vi "PriceData Test.vi"(8 "error in":errorcluster, 11 "IED Test in":refnum<class "IED Test.lvclass">) -> (0 "error out":errorcluster, 2 "Test Result":T1=enum."Success", 3 "IED Test out":refnum<class "IED Test.lvclass">)   [LabVIEW 2018, in "IED Test Framework.lvlib" / "IED Test.lvclass"]
uses:
  IED Test.lvclass
  C:/Program Files (x86)/National Instruments/LabVIEW 2018/vi.lib/ActorFramework/Actor/Actor.lvclass
  C:/Users/Administrator/Desktop/2018LabVIEW EMS/EMS Generic Actor/EMS Generic/EMS Generic.lvclass
  Controls/Test Result.ctl
  <vilib>/ORNL/CSEISMIC DDS/CSEISMIC DDS Base/Data Types/Controls/DeviceClass Selector.ctl
  PriceData Actor/PriceData/PriceData.lvclass
  C:/Users/Administrator/Desktop/2018LabVIEW EMS/IED Actors/Device DDS Communications Framework/Device DDS Communications/Device DDS Communications.lvclass
  <vilib>/ORNL/CSEISMIC DDS/CSEISMIC DDS Base/CSEISMIC DDS.lvclass/CSEISMIC DDS.ctl
  <vilib>/ORNL/CSEISMIC DDS/CSEISMIC DDS Base/Data Types/Controls/DeviceID.ctl
  <vilib>/ActorFramework/Message Enqueuer/Message Enqueuer.lvclass/Message Enqueuer.ctl
  <vilib>/ORNL/CSEISMIC DDS/CSEISMIC DDS Base/Accessors/Write DDS Reference.vi
  <vilib>/ORNL/CSEISMIC DDS/CSEISMIC DDS Base/Accessors/Read DDS Reference.vi
  <vilib>/ActorFramework/Message Enqueuer/Enqueue.vi
  <vilib>/ORNL/CSEISMIC DDS/DDS Writer/DDS Writer.lvclass
  C:/Program Files (x86)/National Instruments/LabVIEW 2018/vi.lib/ORNL/CSEISMIC DDS/CSEISMIC DDS Base/CSEISMIC DDS.lvclass
  <vilib>/ActorFramework/Stop Msg/Stop Msg.lvclass
  C:/Program Files (x86)/National Instruments/LabVIEW 2018/vi.lib/ActorFramework/Message/Message.lvclass
  <vilib>/ORNL/CSEISMIC DDS/CSEISMIC DDS Base/Error Handler.vi
  <vilib>/ActorFramework/Message Priority Queue/Priority Enqueue.vi
  <vilib>/ORNL/CSEISMIC DDS/CSEISMIC DDS Base/CSEISMIC DDS.lvclass
  Device DDS Communications Framework/Device DDS Communications/Device DDS Communications.lvclass
  <vilib>/ActorFramework/Actor/Actor.lvclass
  EMS Generic Actor/EMS Generic/EMS Generic.lvclass
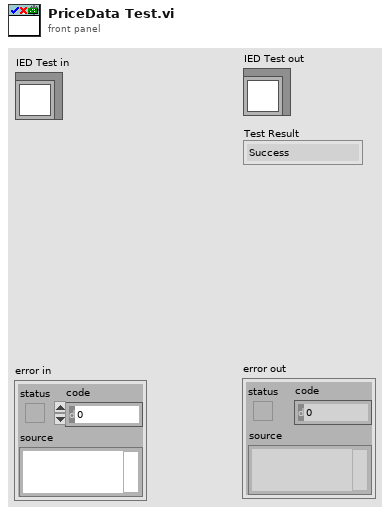
[diagram p1: front panel]
types:
  T1 = typedef "IED Test Framework.lvlib/IED Test.lvclass/Test Result.ctl" = enum16{"Invalid", "Success", "Failure", "Error", "Timeout"}
  T2 = typedef "CSEISMIC DDS.lvlib/CSEISMIC DDS.lvclass/DeviceID.ctl" = string
  T3 = typedef "CSEISMIC DDS.lvlib/CSEISMIC DDS.lvclass/DeviceClass Selector.ctl" = u16
  T4 = typedef "CSEISMIC DDS.lvlib/CSEISMIC DDS.lvclass/PriceData_RealTime.ctl" = cluster{"DeviceID":T2, "t0":dbl, "dt":dbl, "Price":dbl[]}
  T5 = typedef "CSEISMIC DDS.lvlib/CSEISMIC DDS.lvclass/PriceData_Demand.ctl" = cluster{"DeviceID":T2, "DemandCharge ($/kWh)":dbl, "Duration (hours)":dbl}
  T6 = typedef "CSEISMIC DDS.lvlib/CSEISMIC DDS.lvclass/PriceData_Energy.ctl" = cluster{"DeviceID":T2, "EnergyCharge ($/kWh)":dbl}
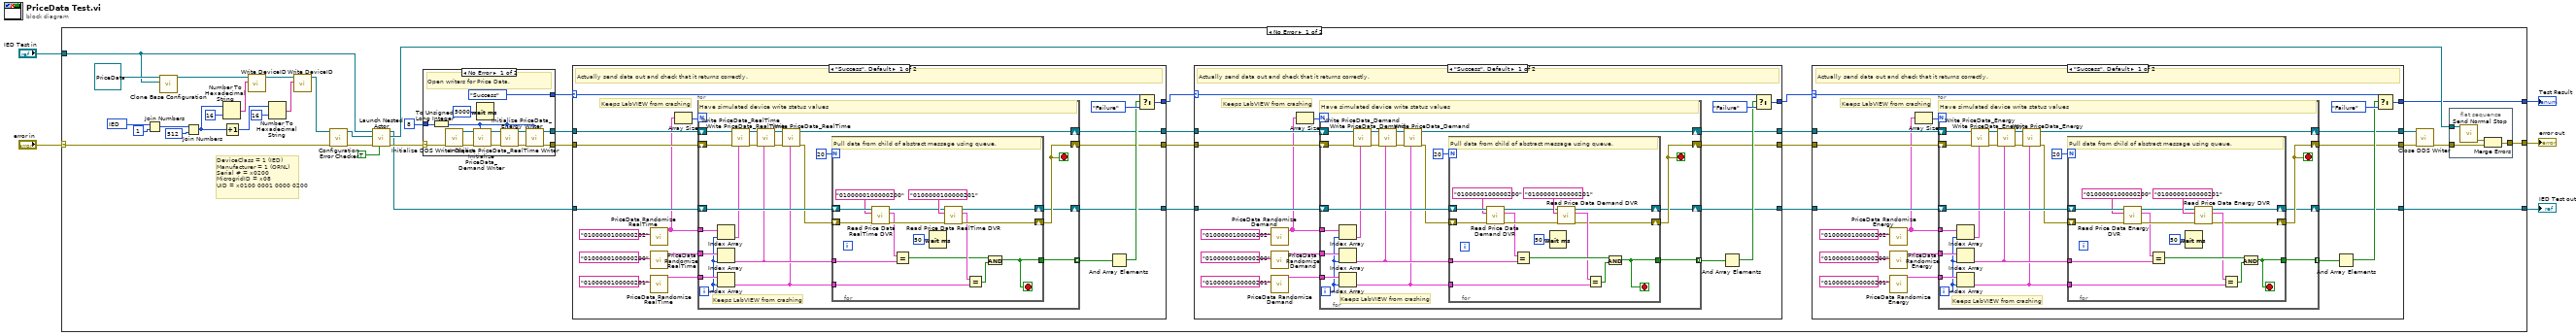
[diagram p0: block diagram]
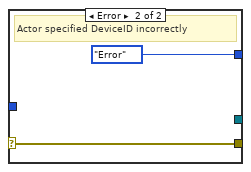
[diagram p5: hidden frame]
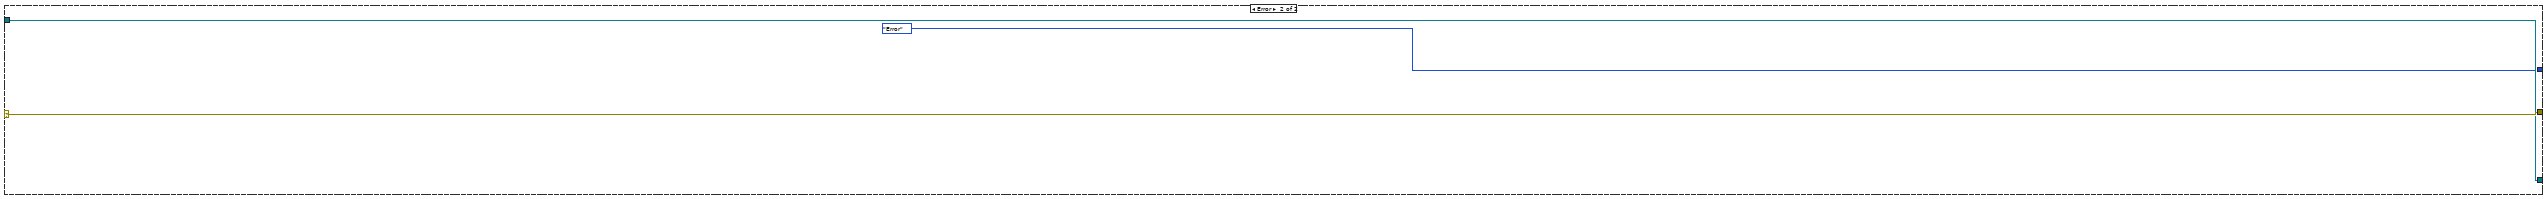
[diagram p6: hidden frame]
diagram:
  n1 = case shown="No Error" "error in" {
    selector: "error in" -> [w41 w241]
    tunnel: [w43 w241] -> w2
    tunnel: [w9 w240] -> w1
    tunnel: "IED Test in" -> [w6 w240]
    tunnel: [w13 Test_Result."Error" ("f")] -> w3
    frame No Error {
      w34 = T3 256 items=["Invalid"=0, "IED"=256, "DER"=512, "Relay"=768, "Meter"=1024, "Load"=1280, "Forecast"=1536, "Price"=1792, "Energy Storage"=513, "PV"=514, "Generator"=515, "Smart Relay"=769, "PCC"=770, "Smart Meter"=1025, "PMU"=1026, "HVAC"=1281] ("DeviceClass")
      # "DeviceClass = 1 (IED)\nManufacturer = 1 (ORNL)\nSerial # = x0200\nMicrogridID = x08\nUID = x0100 0001 0000 0200"
      n2 = Join Numbers(hi=w34, lo=u16 1 ("MicrogridID")) -> ((hi.lo)=w31:u32)
      n3 = call-dynamic "Clone Base Configuration.vi"("Source Object"=w6, "Target Object in"=refnum<class "PriceData.lvclass"> refnum ("PriceData Actor.lvlib:PriceData.lvclass")) -> ("Target Object out"=w7:refnum<class "PriceData.lvclass">)  [unwired: 9 in]
      n4 = Join Numbers(hi=w31, lo=u32 512 ("MicrogridID")) -> ((hi.lo)=w36:u64)
      n5 = Number To Hexadecimal String(1:i16 16 ("width (-)"), 2:w36) -> (0:w29:string)
      n6 = Increment(x=w36) -> (x+1=w38:u64)
      n7 = call-dynamic "Write DeviceID.vi"("DeviceID"=w29, "Device DDS Communications in"=w7) -> ("Device DDS Communications out"=w33:refnum<class "PriceData.lvclass">)  [unwired: 9 in]
      n8 = Number To Hexadecimal String(1:i16 16 ("width (-)"), 2:w38) -> (0:w39:string)
      n9 = call-dynamic "Write DeviceID.vi"("DeviceID"=w39, "Device DDS Communications in"=w33) -> ("Device DDS Communications out"=w19:refnum<class "PriceData.lvclass">)  [unwired: 9 in]
      n10 = call "Configuration Error Checker.vi"("error in"=w41, "Device DDS Communications in"=w19) -> ("error out"=w44:errorcluster, "Device DDS Communications out"=w42:refnum<class "PriceData.lvclass">)  [unwired: 8 in]
      n11 = call <vilib>:"Launch Nested Actor.vi"("Open Actor Core front panel? (F)"=TRUE, "error in (no error)"=w44, "Nested Actor"=w42, "Caller Actor in"=w6) -> ("error out"=w27:errorcluster, "Nested Actor's Enqueuer"=w40:refnum<class "Message Enqueuer.lvclass">, "Caller Actor out"=w10:refnum<class "IED Test.lvclass">)  [unwired: 5 in]
      n12 = case shown="No Error" w27 {
        selector: w27 -> [w234 w238]
        tunnel: [w228 w238] -> w24
        tunnel: u32 8 ("domain id") -> [w236 _]
        tunnel: [Test_Result."Success" ("Test Result in") Test_Result."Error" ("Test Result")] -> w26
        tunnel: [w225 _] -> w25
        frame No Error {
          # "Open writers for Price Data."
          n13 = To Unsigned Long Integer(number=w236) -> (unsigned 32bit integer=w224:u32)
          n14 = call <vilib>:"Initialize DDS Writer Object.vi"("error in"=w234) -> ("error out"=w233:errorcluster, "DDS Writer out"=w232:refnum<class "DDS Writer.lvclass">)  [unwired: 9 in]
          n15 = call <vilib>:"Initialize PriceData_Demand Writer.vi"("MicrogridID"=w224, "error in"=w233, "DDS Writer in"=w232) -> ("error out"=w230:errorcluster, "DDS Writer out"=w231:refnum<class "DDS Writer.lvclass">)  [unwired: 7 in]
          n16 = Wait (ms)(milliseconds to wait=u32 5000) -> ()  [unwired: 1 out]
          n17 = call <vilib>:"Initialize PriceData_Energy Writer.vi"("MicrogridID"=w224, "error in"=w230, "DDS Writer in"=w231) -> ("error out"=w226:errorcluster, "DDS Writer out"=w227:refnum<class "DDS Writer.lvclass">)  [unwired: 7 in]
          n18 = call <vilib>:"Initialize PriceData_RealTime Writer.vi"("MicrogridID"=w224, "error in"=w226, "DDS Writer in"=w227) -> ("error out"=w228:errorcluster, "DDS Writer out"=w225:refnum<class "DDS Writer.lvclass">)  [unwired: 7 in]
        }
        frame Error {
          # "Actor specified DeviceID incorrectly"
        }
      }
      n19 = case shown="\"Success\", Default" w26 {
        selector: w26 -> [w182 w222]
        tunnel: w25 -> [w183 w221]
        tunnel: w10 -> [w177 w220]
        tunnel: w24 -> [w178 w223]
        tunnel: [w180 w222] -> w21
        tunnel: [w176 w223] -> w22
        tunnel: [w174 w221] -> w23
        tunnel: [w167 w220] -> w12
        frame "Success", Default {
          # "Keeps LabVIEW from crashing"
          # "Actually send data out and check that it returns correctly."
          n20 = call "PriceData Randomize RealTime.vi"("DeviceID"=T2 "0100000100000202" ("(hi.lo)")) -> ("ForecastData_Long Array out"=w173:T4[])  [unwired: 10 in]
          n21 = call "PriceData Randomize RealTime.vi"("DeviceID"=T2 "0100000100000200" ("(hi.lo)")) -> ("ForecastData_Long Array out"=w168:T4[])  [unwired: 10 in]
          n22 = call "PriceData Randomize RealTime.vi"("DeviceID"=T2 "0100000100000201" ("(hi.lo)")) -> ("ForecastData_Long Array out"=w169:T4[])  [unwired: 10 in]
          n23 = Array Size(array=w173) -> (size(s)=w175:i32)
          n24 = for {
            N: w175 -> [_]
            shift-right: [w200] -> w174
            shift-left: w183 -> [w203]
            tunnel: w173 -> [w196]
            tunnel: w169 -> [w191]
            tunnel: w168 -> [w192]
            shift-right: [w193] -> w176
            shift-left: w178 -> [w199]
            shift-right: [w187] -> w167
            shift-left: w177 -> [w195]
            tunnel: [w184] -> w166 mode=indexing
            i -> [w189]
            stop <- w193 stop-if-true
            # "Keeps LabVIEW from crashing"
            # "Have simulated device write status values"
            n25 = Index Array(array=w196, index=w189) -> (element=w188:T4)
            n26 = Index Array(array=w192, index=w189) -> (element=w186:T4)
            n27 = Index Array(array=w191, index=w189) -> (element=w185:T4)
            n28 = call <vilib>:"Write PriceData_RealTime.vi"("PriceData_RealTime"=w188, "error in"=w199, "DDS Writer in"=w203) -> ("error out"=w198:errorcluster, "DDS Writer out"=w202:refnum<class "DDS Writer.lvclass">)  [unwired: 7 in]
            n29 = call <vilib>:"Write PriceData_RealTime.vi"("PriceData_RealTime"=w186, "error in"=w198, "DDS Writer in"=w202) -> ("error out"=w197:errorcluster, "DDS Writer out"=w201:refnum<class "DDS Writer.lvclass">)  [unwired: 7 in]
            n30 = call <vilib>:"Write PriceData_RealTime.vi"("PriceData_RealTime"=w185, "error in"=w197, "DDS Writer in"=w201) -> ("error out"=w194:errorcluster, "DDS Writer out"=w200:refnum<class "DDS Writer.lvclass">)  [unwired: 7 in]
            n31 = for {
              N: 20 -> [_]
              shift-right: [w212] -> w193
              shift-left: w194 -> [w218]
              shift-right: [w213] -> w187
              shift-left: w195 -> [w219]
              tunnel: w186 -> [w211]
              tunnel: w185 -> [w209]
              tunnel: [w205] -> w184
              stop <- w205 stop-if-true
              # "Pull data from child of abstract message using queue."
              n32 = call "Read Price Data RealTime DVR.vi"("error in"=w218, "DeviceID"=T2 "0100000100000200" ("(hi.lo)"), "EMS Generic in"=w219) -> ("error out"=w214:errorcluster, "PriceData_RealTime"=w210:T4, "EMS Generic out"=w215:refnum<class "IED Test.lvclass">)  [unwired: 5 in, 1 out]
              n33 = Equal?(x=w210, y=w211) -> (x = y?=w207:bool)
              n34 = Wait (ms)(milliseconds to wait=u32 50) -> ()  [unwired: 1 out]
              n35 = call "Read Price Data RealTime DVR.vi"("error in"=w214, "DeviceID"=T2 "0100000100000201" ("(hi.lo)"), "EMS Generic in"=w215) -> ("error out"=w212:errorcluster, "PriceData_RealTime"=w208:T4, "EMS Generic out"=w213:refnum<class "IED Test.lvclass">)  [unwired: 5 in, 1 out]
              n36 = Equal?(x=w208, y=w209) -> (x = y?=w206:bool)
              n37 = And(x=w207, y=w206) -> (x .and. y?=w205:bool)
            }
          }
          n38 = And Array Elements(Boolean array=w166) -> (logical AND=w179:bool)
          n39 = Select(t=w182, s=w179, f=Test_Result."Failure") -> (s? t:f=w180:T1)
        }
        frame "Error" {
        }
      }
      n40 = case shown="\"Success\", Default" w21 {
        selector: w21 -> [w124 w164]
        tunnel: w23 -> [w125 w163]
        tunnel: w12 -> [w119 w162]
        tunnel: w22 -> [w120 w165]
        tunnel: [w122 w164] -> w16
        tunnel: [w118 w165] -> w17
        tunnel: [w116 w163] -> w18
        tunnel: [w108 w162] -> w11
        frame "Success", Default {
          # "Keeps LabVIEW from crashing"
          # "Actually send data out and check that it returns correctly."
          n41 = call "PriceData Randomize Demand.vi"("DeviceID"=T2 "0100000100000202" ("(hi.lo)")) -> ("PriceData_Demand Array out"=w115:T5[])  [unwired: 10 in]
          n42 = call "PriceData Randomize Demand.vi"("DeviceID"=T2 "0100000100000200" ("(hi.lo)")) -> ("PriceData_Demand Array out"=w110:T5[])  [unwired: 10 in]
          n43 = call "PriceData Randomize Demand.vi"("DeviceID"=T2 "0100000100000201" ("(hi.lo)")) -> ("PriceData_Demand Array out"=w111:T5[])  [unwired: 10 in]
          n44 = Array Size(array=w115) -> (size(s)=w117:i32)
          n45 = for {
            N: w117 -> [_]
            shift-right: [w142] -> w116
            shift-left: w125 -> [w145]
            tunnel: w115 -> [w138]
            tunnel: w111 -> [w133]
            tunnel: w110 -> [w134]
            shift-right: [w135] -> w118
            shift-left: w120 -> [w141]
            shift-right: [w127] -> w108
            shift-left: w119 -> [w137]
            tunnel: [w126] -> w109 mode=indexing
            i -> [w131]
            stop <- w135 stop-if-true
            # "Keeps LabVIEW from crashing"
            # "Have simulated device write status values"
            n46 = Index Array(array=w138, index=w131) -> (element=w130:T5)
            n47 = Index Array(array=w134, index=w131) -> (element=w129:T5)
            n48 = Index Array(array=w133, index=w131) -> (element=w128:T5)
            n49 = call <vilib>:"Write PriceData_Demand.vi"("PriceData_Demand"=w130, "error in"=w141, "DDS Writer in"=w145) -> ("error out"=w140:errorcluster, "DDS Writer out"=w144:refnum<class "DDS Writer.lvclass">)  [unwired: 7 in]
            n50 = call <vilib>:"Write PriceData_Demand.vi"("PriceData_Demand"=w129, "error in"=w140, "DDS Writer in"=w144) -> ("error out"=w139:errorcluster, "DDS Writer out"=w143:refnum<class "DDS Writer.lvclass">)  [unwired: 7 in]
            n51 = call <vilib>:"Write PriceData_Demand.vi"("PriceData_Demand"=w128, "error in"=w139, "DDS Writer in"=w143) -> ("error out"=w136:errorcluster, "DDS Writer out"=w142:refnum<class "DDS Writer.lvclass">)  [unwired: 7 in]
            n52 = for {
              N: 20 -> [_]
              shift-right: [w148] -> w135
              shift-left: w136 -> [w157]
              shift-right: [w147] -> w127
              shift-left: w137 -> [w158]
              tunnel: w129 -> [w151]
              tunnel: w128 -> [w150]
              tunnel: [w146] -> w126
              stop <- w146 stop-if-true
              # "Pull data from child of abstract message using queue."
              n53 = call "Read Price Data Demand DVR.vi"("error in"=w157, "DeviceID"=T2 "0100000100000200" ("(hi.lo)"), "EMS Generic in"=w158) -> ("error out"=w153:errorcluster, "PriceData_Demand"=w152:T5, "EMS Generic out"=w154:refnum<class "IED Test.lvclass">)  [unwired: 5 in, 1 out]
              n54 = Equal?(x=w152, y=w151) -> (x = y?=w159:bool)
              n55 = Wait (ms)(milliseconds to wait=u32 50) -> ()  [unwired: 1 out]
              n56 = call "Read Price Data Demand DVR.vi"("error in"=w153, "DeviceID"=T2 "0100000100000201" ("(hi.lo)"), "EMS Generic in"=w154) -> ("error out"=w148:errorcluster, "PriceData_Demand"=w149:T5, "EMS Generic out"=w147:refnum<class "IED Test.lvclass">)  [unwired: 5 in, 1 out]
              n57 = Equal?(x=w149, y=w150) -> (x = y?=w160:bool)
              n58 = And(x=w159, y=w160) -> (x .and. y?=w146:bool)
            }
          }
          n59 = And Array Elements(Boolean array=w109) -> (logical AND=w121:bool)
          n60 = Select(t=w124, s=w121, f=Test_Result."Failure") -> (s? t:f=w122:T1)
        }
        frame "Error" {
        }
      }
      n61 = case shown="\"Success\", Default" w16 {
        selector: w16 -> [w62 w102]
        tunnel: w18 -> [w63 w101]
        tunnel: w11 -> [w57 w100]
        tunnel: w17 -> [w58 w103]
        tunnel: [w60 w102] -> w13
        tunnel: [w56 w103] -> w14
        tunnel: [w54 w101] -> w15
        tunnel: [w46 w100] -> w9
        frame "Success", Default {
          # "Keeps LabVIEW from crashing"
          # "Actually send data out and check that it returns correctly."
          n62 = call "PriceData Randomize Energy.vi"("DeviceID"=T2 "0100000100000202" ("(hi.lo)")) -> ("PriceData_Energy Array out"=w53:T6[])  [unwired: 10 in]
          n63 = call "PriceData Randomize Energy.vi"("DeviceID"=T2 "0100000100000200" ("(hi.lo)")) -> ("PriceData_Energy Array out"=w48:T6[])  [unwired: 10 in]
          n64 = call "PriceData Randomize Energy.vi"("DeviceID"=T2 "0100000100000201" ("(hi.lo)")) -> ("PriceData_Energy Array out"=w49:T6[])  [unwired: 10 in]
          n65 = Array Size(array=w53) -> (size(s)=w55:i32)
          n66 = for {
            N: w55 -> [_]
            shift-right: [w80] -> w54
            shift-left: w63 -> [w83]
            tunnel: w53 -> [w76]
            tunnel: w49 -> [w71]
            tunnel: w48 -> [w72]
            shift-right: [w73] -> w56
            shift-left: w58 -> [w79]
            shift-right: [w67] -> w46
            shift-left: w57 -> [w75]
            tunnel: [w64] -> w47 mode=indexing
            i -> [w69]
            stop <- w73 stop-if-true
            # "Keeps LabVIEW from crashing"
            # "Have simulated device write status values"
            n67 = Index Array(array=w76, index=w69) -> (element=w68:T6)
            n68 = Index Array(array=w72, index=w69) -> (element=w66:T6)
            n69 = Index Array(array=w71, index=w69) -> (element=w65:T6)
            n70 = call <vilib>:"Write PriceData_Energy.vi"("PriceData_Energy"=w68, "error in"=w79, "DDS Writer in"=w83) -> ("error out"=w78:errorcluster, "DDS Writer out"=w82:refnum<class "DDS Writer.lvclass">)  [unwired: 7 in]
            n71 = call <vilib>:"Write PriceData_Energy.vi"("PriceData_Energy"=w66, "error in"=w78, "DDS Writer in"=w82) -> ("error out"=w77:errorcluster, "DDS Writer out"=w81:refnum<class "DDS Writer.lvclass">)  [unwired: 7 in]
            n72 = call <vilib>:"Write PriceData_Energy.vi"("PriceData_Energy"=w65, "error in"=w77, "DDS Writer in"=w81) -> ("error out"=w74:errorcluster, "DDS Writer out"=w80:refnum<class "DDS Writer.lvclass">)  [unwired: 7 in]
            n73 = for {
              N: 20 -> [_]
              shift-right: [w87] -> w73
              shift-left: w74 -> [w95]
              shift-right: [w88] -> w67
              shift-left: w75 -> [w96]
              tunnel: w66 -> [w86]
              tunnel: w65 -> [w85]
              tunnel: [w84] -> w64
              stop <- w84 stop-if-true
              # "Pull data from child of abstract message using queue."
              n74 = call "Read Price Data Energy DVR.vi"("error in"=w95, "DeviceID"=T2 "0100000100000200" ("(hi.lo)"), "EMS Generic in"=w96) -> ("error out"=w91:errorcluster, "PriceData_Energy"=w90:T6, "EMS Generic out"=w92:refnum<class "IED Test.lvclass">)  [unwired: 5 in, 1 out]
              n75 = Equal?(x=w90, y=w86) -> (x = y?=w99:bool)
              n76 = Wait (ms)(milliseconds to wait=u32 50) -> ()  [unwired: 1 out]
              n77 = call "Read Price Data Energy DVR.vi"("error in"=w91, "DeviceID"=T2 "0100000100000201" ("(hi.lo)"), "EMS Generic in"=w92) -> ("error out"=w87:errorcluster, "PriceData_Energy"=w89:T6, "EMS Generic out"=w88:refnum<class "IED Test.lvclass">)  [unwired: 5 in, 1 out]
              n78 = Equal?(x=w89, y=w85) -> (x = y?=w98:bool)
              n79 = And(x=w99, y=w98) -> (x .and. y?=w84:bool)
            }
          }
          n80 = And Array Elements(Boolean array=w47) -> (logical AND=w59:bool)
          n81 = Select(t=w62, s=w59, f=Test_Result."Failure") -> (s? t:f=w60:T1)
        }
        frame "Error" {
        }
      }
      n82 = call <vilib>:"Close DDS Writer.vi"("error in"=w14, "DDS Writer in"=w15) -> ("error out"=w20:errorcluster)  [unwired: 9 in]
      n83 = flat-sequence {
        tunnel: w40 -> [w107]
        tunnel: [w105] -> w43
        tunnel: w20 -> [w104]
        frame #0 {
          n84 = call <vilib>:"Send Normal Stop.vi"("Message Enqueuer"=w107) -> ("error out"=w106:errorcluster)  [unwired: 10 in]
          n85 = Merge Errors(w106, w104) -> (w105:errorcluster)
        }
      }
    }
    frame Error {
    }
  }
  "error out" <- w2
  "IED Test out" <- w1
  "Test Result" <- w3
